vi "Read Site Info.vi"(8 "error in (no error)":errorcluster, 11 "WebView2 Control in":refnum<class "WebView2 Control.lvclass">) -> (0 "error out":errorcluster, 2 "Site Info":T1, 3 "WebView2 Control out":refnum<class "WebView2 Control.lvclass">)   [LabVIEW 2020, in "WebView2.lvlib" / "WebView2 Control.lvclass"]
uses:
  WebView2 Control.lvclass
  WebView2 Control.lvclass/WebView2 Control.ctl
  C:/Users/Simon/Documents/GitHub/LV-WebView2/Source/Libs/Microsoft.Web.WebView2.Core.dll
  Libs/Microsoft.Web.WebView2.Core.dll
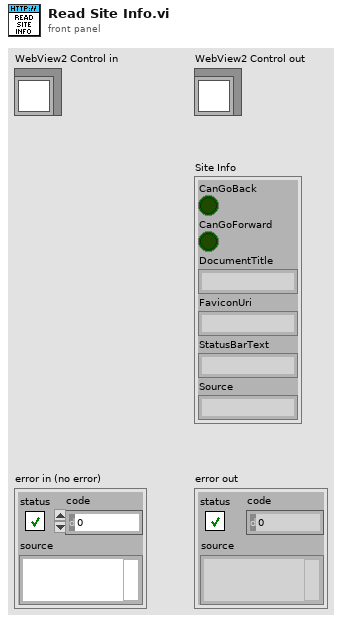
[diagram p1: front panel]
types:
  T1 = cluster{"CanGoBack":bool, "CanGoForward":bool, "DocumentTitle":string, "FaviconUri":string, "StatusBarText":string, "Source":string}
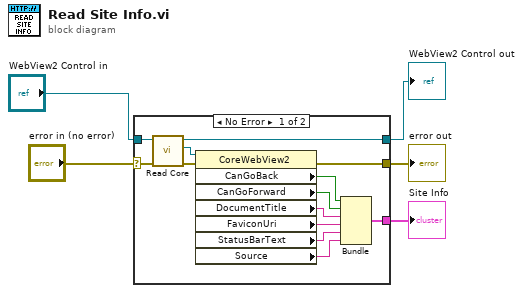
[diagram p0: block diagram]
diagram:
  n1 = case shown="No Error" "error in (no error)" {
    selector: "error in (no error)" -> [w7 w20]
    tunnel: [w12 w20] -> w4
    tunnel: [w9 w19] -> w2
    tunnel: "WebView2 Control in" -> [w10 w19]
    tunnel: [w11 _] -> w1
    frame No Error {
      n2 = call "Read Core.vi"("error in (no error)"=w7, "WebView2.lvlib:WebView2 Control.lvclass"=w10) -> ("error out"=w6:errorcluster, "Webview2 Core"=w8:refnum<k24>, "WebView2.lvlib:WebView2 Control.lvclass"=w9:refnum<class "WebView2 Control.lvclass">)  [unwired: 7 in]
      n3 = property class="CoreWebView2"(reference=w8, error in=w6) -> (error out=w12:errorcluster, "CanGoBack"=w18:bool, "CanGoForward"=w17:bool, "DocumentTitle"=w16:string, "FaviconUri"=w15:string, "StatusBarText"=w14:string, "Source"=w13:string)  [unwired: 1 out]
      n4 = Bundle("CanGoBack"=w18, "CanGoForward"=w17, "DocumentTitle"=w16, "FaviconUri"=w15, "StatusBarText"=w14, "Source"=w13) -> (w11:T1)  [unwired: 1 in]
    }
    frame Error {
    }
  }
  "error out" <- w4
  "WebView2 Control out" <- w2
  "Site Info" <- w1
